vi "Control de Temperatura Max-Min.vi"() -> ()   [LabVIEW 2019]
panel:
  in  "Decremento T":dbl(knob) scale=0.0..10.0
  in  "Incremento T":dbl(knob) scale=0.0..10.0
  out "Decremento":bool
  out "Incremento":bool
  in  "Selector":bool
  in  "RATA DE T (°C/Seg)":dbl(knob) scale=0.0..10.0
  in  "Temp Mín":dbl
  in  "Temp Máx":dbl
  out "Sensor de Temperatura °C":dbl(slide) scale=0.0..200.0
  # "INCREMENTAR"
  # "DECREMENTAR"
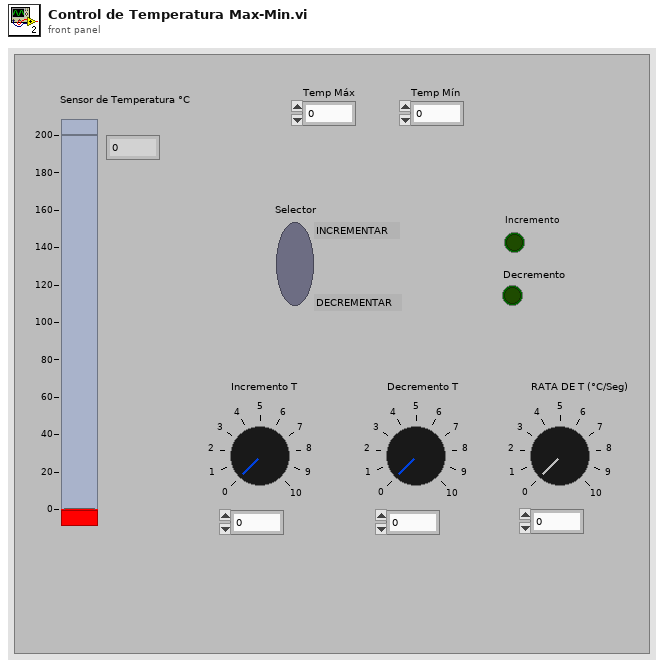
[diagram p1: front panel]
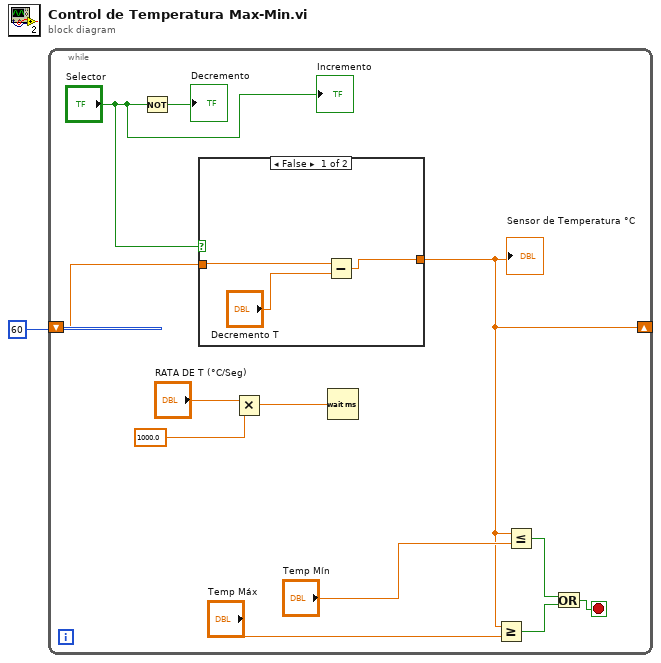
[diagram p0: block diagram]
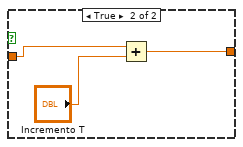
[diagram p2: hidden frame]
diagram:
  n1 = while {
    shift-right: [w4] -> _
    shift-left: 60 -> [w8]
    stop <- w13 stop-if-true
    n2 = Not(x="Selector") -> (.not. x?=→"Decremento":bool)
    n3 = case shown="False" "Selector" {
      tunnel: w8 -> [w14 w18]
      tunnel: [w16 w19] -> w4
      frame False {
        n4 = Subtract(x=w14, y="Decremento T") -> (x-y=w16:dbl)
      }
      frame True {
        n5 = Add(x=w18, y="Incremento T") -> (x+y=w19:dbl)
      }
    }
    "Sensor de Temperatura °C" <- w4
    n6 = Multiply(x="RATA DE T (°C/Seg)", y=1000.0) -> (x*y=w5:dbl)
    n7 = Wait (ms)(milliseconds to wait=w5) -> ()  [unwired: 1 out]
    n8 = Greater Or Equal?(x=w4, y="Temp Máx") -> (x >= y?=w11:bool)
    n9 = Less Or Equal?(x=w4, y="Temp Mín") -> (x <= y?=w10:bool)
    n10 = Or(x=w10, y=w11) -> (x .or. y?=w13:bool)
    "Incremento" <- "Selector"
  }
